vi "LEBITVacuum.PubMonServices.vi"(0 "i ref in":refnum<vi>, 2 "i attribute in":T1={"setValuePLC"=[], "nickNames"=[], "setValuePLCServiceID"=[], "monValuePLC"=[], "SetValueServiceID"=[], "MonValueServiceID"=[], "SetValue"=[], "AllPLCValues"=[], "CondSpecial2DArray"=[], "CondSpecialIndex"=[], "ReasonForLocking"="", "ReasonForLockingID"=0, "enableValuePLC"=[], "OverwriteCloseSafetyPLC"=[], "OverwriteOpenSafetyPLC"=[], "OverwriteCloseSafetyPLCServiceID"=[], "OverwriteOpenSafetyPLCServiceID"=[], "MKS Address Array"=[], "MKS MeasurementServiceID"=[], "MKS Measurement"=[], "CRYO Measurement"=[], "CRYO MeasurementServiceID"=[], "Special"=[], "Start Date"="", "MKS VISA resource"="COM13", "CRYO VISA resource"="COM13"}, 5 "error in":errorcluster) -> (14 "i ref out":refnum<vi>, 16 "i attribute out":T1={"setValuePLC"=[], "nickNames"=[], "setValuePLCServiceID"=[], "monValuePLC"=[], "SetValueServiceID"=[], "MonValueServiceID"=[], "SetValue"=[], "AllPLCValues"=[], "CondSpecial2DArray"=[], "CondSpecialIndex"=[], "ReasonForLocking"="", "ReasonForLockingID"=0, "enableValuePLC"=[], "OverwriteCloseSafetyPLC"=[], "OverwriteOpenSafetyPLC"=[], "OverwriteCloseSafetyPLCServiceID"=[], "OverwriteOpenSafetyPLCServiceID"=[], "MKS Address Array"=[], "MKS MeasurementServiceID"=[], "MKS Measurement"=[], "CRYO Measurement"=[], "CRYO MeasurementServiceID"=[], "Special"=[], "Start Date"="", "MKS VISA resource"="COM13", "CRYO VISA resource"="COM13"}, 17 "MonValueServiceID":i32[](array[numeric]), 19 "error out":errorcluster)   [LabVIEW 2014, in "LEBITVacuum.lvlib"]
uses:
  LEBITVacuum.lvlib
  LEBITVacuum.i attribute.ctl
  CSlibraries/UtilityLib/UtilityLib.valueStatus.ctl
  CSlibraries/UtilityLib/UtilityLib.lvlib
  CSCore/CSSystem/CoreLib/CoreLib.lvlib
  CSlibraries-extern/DimLVEvent/LVDimInterface/LVDimInterface.lvlib
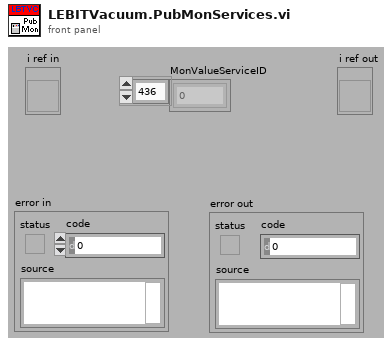
[diagram p1: front panel]
types:
  T1 = typedef "LEBITVacuum.lvlib/LEBITVacuum.i attribute.ctl" = cluster{"setValuePLC":string[], "nickNames":string[], "setValuePLCServiceID":i32[], "monValuePLC":string[], "SetValueServiceID":i32[], "MonValueServiceID":i32[], "SetValue":i16[], "AllPLCValues":string[], "CondSpecial2DArray":string[][], "CondSpecialIndex":i32[], "ReasonForLocking":string, "ReasonForLockingID":i32, "enableValuePLC":string[], "OverwriteCloseSafetyPLC":string[], "OverwriteOpenSafetyPLC":string[], "OverwriteCloseSafetyPLCServiceID":i32[], "OverwriteOpenSafetyPLCServiceID":i32[], "MKS Address Array":i32[][], "MKS MeasurementServiceID":i32[], "MKS Measurement":string[], "CRYO Measurement":string[][], "CRYO MeasurementServiceID":i32[], "Special":string[], "Start Date":string, "MKS VISA resource":refnum<visa-resource-name>, "CRYO VISA resource":refnum<visa-resource-name>}
  T2 = typedef "UtilityLib.lvlib/UtilityLib.valueStatus.ctl" = enum16{"no info available", "stand by/off", "on", "warning", "alarm/malfunction", "not implemented", "user action required", "important information", "system default", "control default", "indicator default", "button default"}
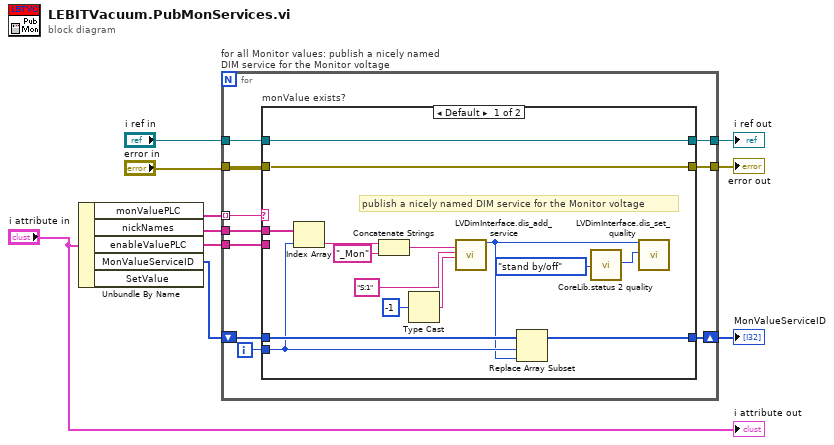
[diagram p0: block diagram]
diagram:
  n1 = Unbundle By Name("i attribute in") -> ("monValuePLC"=w3:string[], "nickNames"=w6:string[], "enableValuePLC"=w1:string[], "MonValueServiceID"=w2:i32[])  [unwired: 1 out]
  n2 = for "for all Monitor values: publish a nicely named DIM service for the Monitor voltage" {
    tunnel: w3 -> [w20] mode=indexing
    tunnel: w6 -> [w19]
    shift-right: [w16] -> w9
    shift-left: w2 -> [w17]
    tunnel: "i ref in" -> [w15]
    tunnel: "error in" -> [w14]
    tunnel: [w13] -> w8
    tunnel: [w12] -> w7
    tunnel: w1 -> [w11]
    i -> [w18]
    n3 = case "monValue exists?" shown="Default" w20 {
      tunnel: w19 -> [w35 _]
      tunnel: w18 -> [w33 _]
      tunnel: w17 -> [w34 w38]
      tunnel: [w32 w38] -> w16
      tunnel: w15 -> [w31 w37]
      tunnel: w14 -> [w30 w36]
      tunnel: [w30 w36] -> w13
      tunnel: [w31 w37] -> w12
      tunnel: w11 -> [_ _]
      frame Default {
        # "publish a nicely named DIM service for the Monitor voltage"
        n4 = Index Array(array=w35, index=w33) -> (element=w22:string)
        n5 = Concatenate Strings(w22, "_Mon" ("string")) -> (w28:string)
        n6 = Type Cast(x=i16 -1) -> (*(type *) &x=w27:string)  [unwired: 1 in]
        n7 = call "LVDimInterface.dis_add_service.vi"("serviceName"=w28, "typeDescriptor"="S:1", "data"=w27) -> ("my_serviceID"=w23:i32)  [unwired: 15 in, 1 out]
        n8 = Replace Array Subset(array=w34, new element=w23, index=w33) -> (w32:i32[])
        n9 = call "CoreLib.status 2 quality.vi"("valueStatus"=UtilityLib.valueStatus."stand by/off") -> ("quality"=w25:i32)  [unwired: 18 in]
        n10 = call "LVDimInterface.dis_set_quality.vi"("my_serviceID"=w23, "quality"=w25) -> ()  [unwired: 16 in, 2 out]
      }
      frame "" {
      }
    }
  }
  "MonValueServiceID" <- w9
  "error out" <- w8
  "i ref out" <- w7
  "i attribute out" <- "i attribute in"
